vi "Private Test.vi"() -> ()   [LabVIEW 2017, in "Private Test.lvlib"]
uses:
  Private Test.lvlib
  <vilib>/PNR/Transparent Assertions/Transparent Assertions/Assertions/Assertions.lvlib
panel:
  out "error out":errorcluster
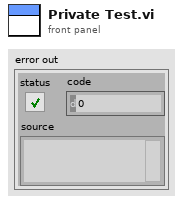
[diagram p1: front panel]
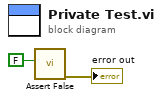
[diagram p0: block diagram]
diagram:
  n1 = call <vilib>:"Assert False.vi"("Condition"=FALSE) -> ("error out"=→"error out":errorcluster)  [unwired: 10 in]
